vi "Actor Core.vi"(8 "error in":errorcluster, 11 "Nested in":refnum<class "Displayer.lvclass">) -> (0 "error out":errorcluster, 3 "Actor out":refnum<class "Actor.lvclass">)   [LabVIEW 2020, in "Displayer.lvlib" / "Displayer.lvclass"]
doc: "(<B>Filename</B>: Actor Framework.lvlib:Actor.lvclass:Actor Core.vi)\n\nReceives messages to the actor, reacts to them, and initiates any error handling that may shut the actor down.\n\nDescendant classes may override this VI to append parallel tasks for the actor to complete while it handles messages. Overrides use the Call Parent Method node."
uses:
  Displayer.lvclass
  <vilib>/ActorFramework/Actor/Actor.lvclass
  <vilib>/ActorFramework/Stop Msg/Stop Msg.lvclass
  C:/Program Files/National Instruments/LabVIEW 2020/vi.lib/ActorFramework/Actor/Actor.lvclass
panel:
  out "String":string
  in  "Boolean":bool
  in  "Numeric":dbl
  # "Demo Controller"
  # "Place your own control/indicator here"
  # "Events for UI Actor Indicators, add Event support in a click away!"
  # "https://forums.ni.com/t5/Actor-Framework-Documents/Events-for-UI-Actor-Indicators/ta-p/3869260?profile.language=en"
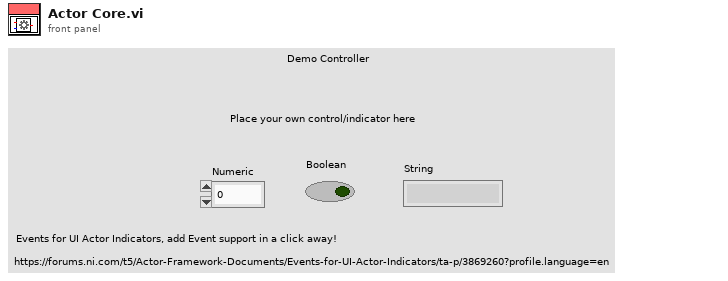
[diagram p1: front panel]
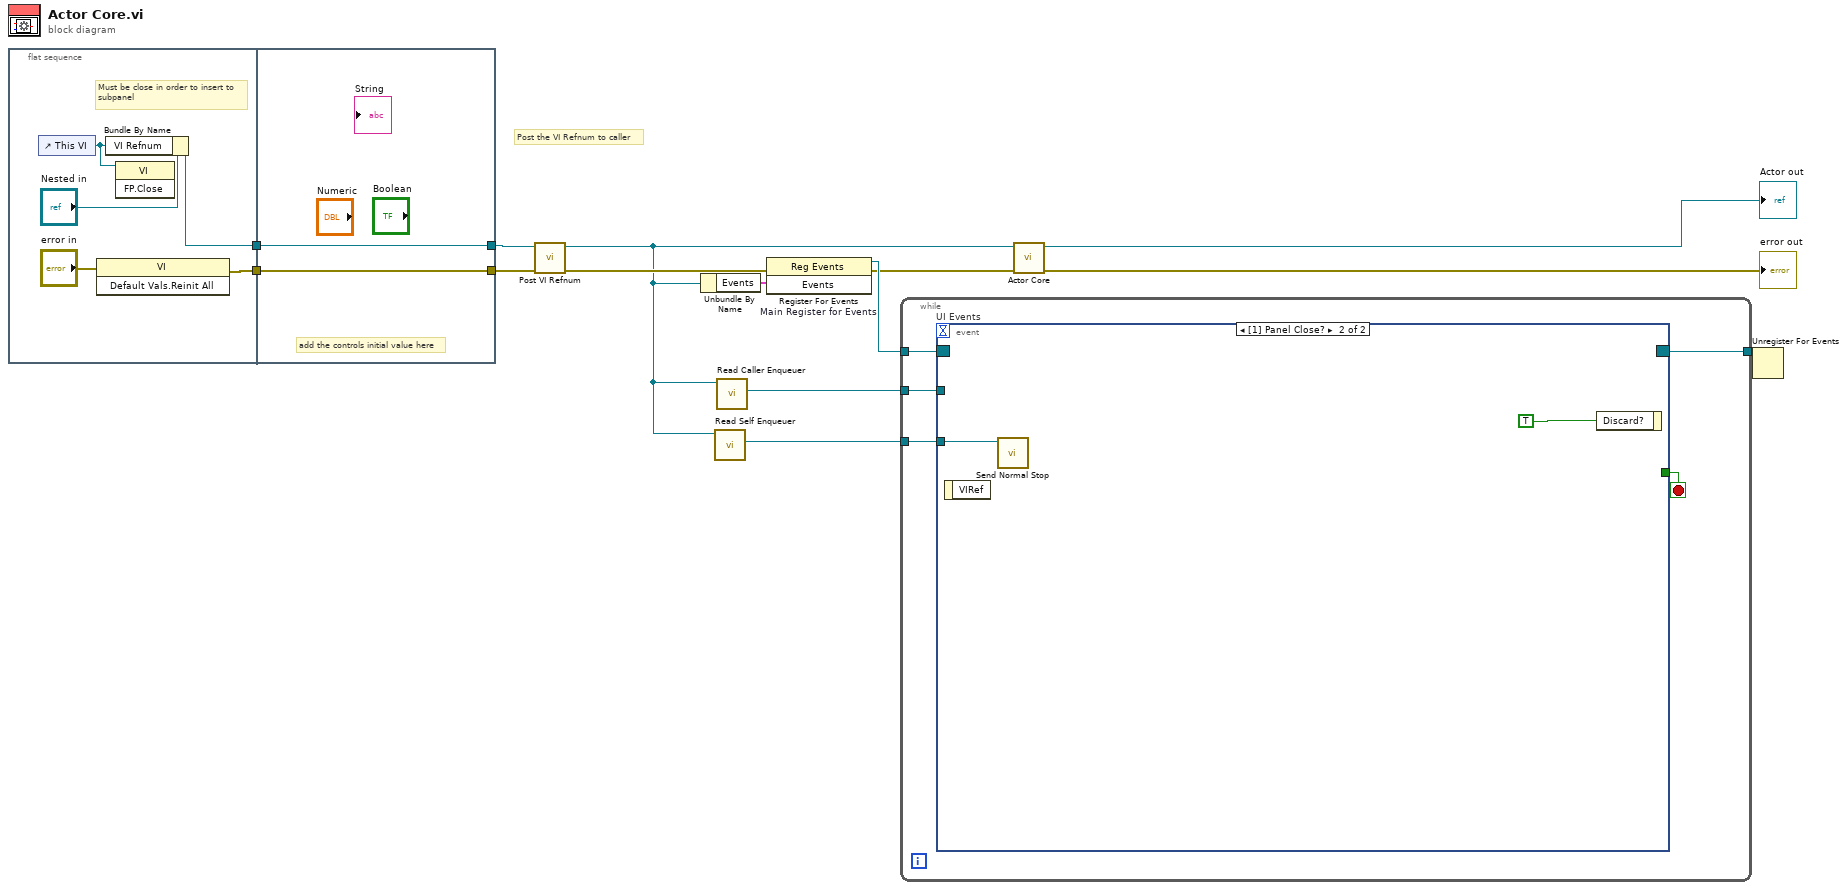
[diagram p0: block diagram]
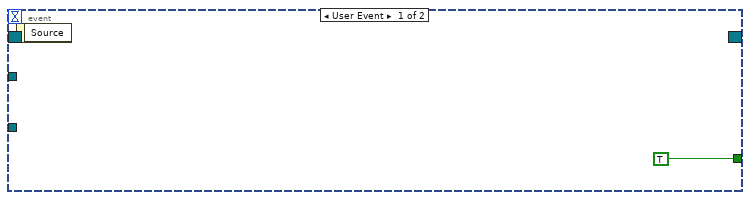
[diagram p2: hidden frame]
diagram:
  # "Post the VI Refnum to caller"
  n1 = flat-sequence {
    tunnel: [w17] -> w6
    tunnel: [w16] -> w5
    tunnel: [w20] -> w3
    tunnel: [w21] -> w7
    tunnel: w6 -> [w21]
    tunnel: w5 -> [w20]
    frame #0 {
      # "Must be close in order to insert to\nsubpanel"
      n2 = control-ref of="This VI"() -> (w15:refnum<vi>)
      n3 = invoke class="VI" method="Default Vals.Reinit All"(error in="error in") -> (error out=w17:errorcluster)  [unwired: 2 in, 2 out]
      n4 = Bundle By Name(cluster="Nested in", "VI Refnum"=w15) -> (w16:refnum<class "Displayer.lvclass">)
      n5 = invoke class="VI" method="FP.Close"(reference=w15) -> ()  [unwired: 2 in, 3 out]
    }
    frame #1 {
      # "add the controls initial value here"
    }
  }
  n6 = call-dynamic "Post VI Refnum.vi"("error in (no error)"=w7, "Controller Template in"=w3) -> ("error out"=w4:errorcluster, "Controller Template out"=w2:refnum<class "Displayer.lvclass">)  [unwired: 8 in]
  n7 = Unbundle By Name(w2) -> ("Events"=w11:cluster{"Stop":refnum<user-event>})
  n8 = call <vilib>:"Read Self Enqueuer.vi"("Actor"=w2) -> ("Self Enqueuer"=w9:refnum<class "Message Enqueuer.lvclass">)  [unwired: 10 in]
  n9 = call <vilib>:"Read Caller Enqueuer.vi"("Actor"=w2) -> ("Caller Enqueuer"=w1:refnum<class "Message Enqueuer.lvclass">)  [unwired: 10 in]
  n10 = register-events "Main Register for Events"(error in=w4, w11) -> (reference out=w12:refnum<event-registration>, error out=w8:errorcluster)  [unwired: 1 in]
  n11 = while {
    tunnel: w12 -> [w26]
    tunnel: [w24] -> w10
    tunnel: w9 -> [w23]
    tunnel: w1 -> [w22]
    stop <- w25 stop-if-true
    n12 = event "UI Events" shown="[1] Panel Close?" {
      selector: w26 -> [_ _]
      dyn-events: [_ _] -> w24
      timeout: _ -> [_ _]
      tunnel: [TRUE _] -> w25
      tunnel: w23 -> [_ w28]
      tunnel: w22 -> [_ _]
      event User Event {
        n13 = event-data() -> ()  [unwired: 1 in, 1 out]
      }
      event Panel Close? {
        n14 = event-data() -> ()  [unwired: 1 in, 1 out]
        n15 = call <vilib>:"Send Normal Stop.vi"("Message Enqueuer"=w28) -> ()  [unwired: 10 in, 1 out]
        n16 = event-data("Discard?"=TRUE) -> ()  [unwired: 1 in, 1 out]
      }
    }
  }
  n17 = call-parent "Actor Core.vi"("error in"=w8, "Actor in"=w2) -> ("error out"=→"error out":errorcluster, "Actor out"=→"Actor out":refnum<class "Actor.lvclass">)  [unwired: 8 in]
  n18 = Unregister For Events(event registration refnum=w10) -> ()  [unwired: 1 in, 1 out]
